vi "CRYInitialize Menu.vi"   [LabVIEW 2013]
uses:
  <vilib>/Utility/miscctls.llb/LVMenuShortCut.ctl
  SubVI/CRYMain Sub Window Global.vi
panel:
  # "Menu Initialize"
types:
  T1 = typedef "LVMenuShortCut.ctl" = cluster{"Include Shift Key?":bool, "Include Ctrl Key?":bool, "Shortcut Key":string}
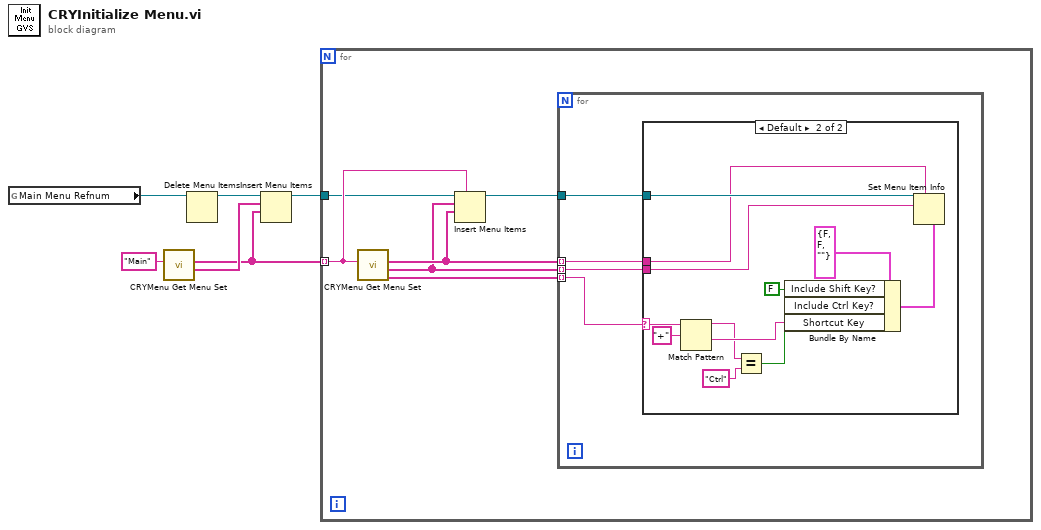
[diagram p0: block diagram]
diagram:
  n1 = global read "CRYMain Sub Window Global.vi" "Main Menu Refnum"() -> (w1:refnum<k9>)
  n2 = call "CRYMenu Get Menu Set.vi"("sMenuTag"="Main") -> ("sMultibyte_Out"=w5:string[], "sID_Out"=w3:string[])  [unwired: 7 in, 2 out]
  n3 = Delete Menu Items(9:w1) -> (3:w4:refnum<k9>)  [unwired: 3 in, 1 out]
  n4 = Insert Menu Items(7:w3, 8:w5, 9:w4) -> (3:w2:refnum<k9>)  [unwired: 3 in, 2 out]
  n5 = for {
    tunnel: w3 -> [w12] mode=indexing
    tunnel: w2 -> [w11]
    n6 = call "CRYMenu Get Menu Set.vi"("sMenuTag"=w12) -> ("sShortcut_Out"=w10:string[], "sMultibyte_Out"=w7:string[], "sID_Out"=w8:string[])  [unwired: 7 in, 1 out]
    n7 = Insert Menu Items(5:w12, 7:w8, 8:w7, 9:w11) -> (3:w9:refnum<k9>)  [unwired: 2 in, 2 out]
    n8 = for {
      tunnel: w10 -> [w13] mode=indexing
      tunnel: w9 -> [w16]
      tunnel: w8 -> [w15] mode=indexing
      tunnel: w7 -> [w14] mode=indexing
      n9 = case shown="Default" w13 {
        selector: w13 -> [_ w25]
        tunnel: w16 -> [_ w28]
        tunnel: w15 -> [_ w27]
        tunnel: w14 -> [_ w26]
        frame "" {
        }
        frame Default {
          n10 = Match Pattern(string=w25, regular expression="+") -> (before substring=w19:string, after substring=w21:string)  [unwired: 1 in, 2 out]
          n11 = Equal?(x=w19, y="Ctrl" ("before substring")) -> (x = y?=w17:bool)
          n12 = Bundle By Name(cluster=T1 {"Include Shift Key?"=FALSE, "Include Ctrl Key?"=FALSE, "Shortcut Key"=""} ("short cut"), "Include Shift Key?"=FALSE, "Include Ctrl Key?"=w17, "Shortcut Key"=w21) -> (w20:T1)
          n13 = Set Menu Item Info(4:w20, 7:w27, 10:w26, 11:w28) -> ()  [unwired: 3 in, 2 out]
        }
      }
    }
  }
